vi "master_python_v1.0.vi"() -> ()   [LabVIEW 2026]
uses:
  Nanostage/Madlib.dll
  <vilib>/Utility/error.llb/DialogType.ctl
  <vilib>/DAQmx/read.llb/DAQmx Read (Analog 1D Wfm NChan NSamp).vi
  <vilib>/DAQmx/read.llb/DAQmx Read (Analog 1D Wfm NChan NSamp Duration).vi
  <vilib>/DAQmx/write.llb/DAQmx Write (Analog 2D DBL NChan NSamp).vi
  <vilib>/Utility/inputDevices.llb/keyboardAcquire.vi
panel:
  out "PID output":dbl format="%.2f"
  out "Setpoint":dbl
  in  "PID gains":T1={"proportional gain (Kc)"=0.5, "integral time (Ti, min)"=0.0, "derivative time (Td, min)"=0.0} {"derivative time (Td, min)" min=-1e-18 max=1000000000000000.0 step=1e-05 format="%.3f"; "integral time (Ti, min)" min=-1e-18 step=1e-05 format="%.6f"; "proportional gain (Kc)" min=-1e-18 step=1e-05 format="%.5f"}
  in  "output range":cluster{"output high":dbl, "output low":dbl}={"output high"=0.1, "output low"=-0.1} {"output low" format="%.2f"; "output high" format="%.2f"}
  in  "dt (s)":dbl=-1.0 format="%.3f"
  out "QPD":dbl
  out "Pos 0":dbl
  in  "Comment":string
  out "loop iteration":i32
  out "x start":dbl
  out "y start":dbl
  out "z start":dbl
  out "start iteration":dbl
  out "data":waveform(dbl)[](array[waveform])
  out "Numeric 2":i32
  out "Numeric":i32
  out "stop Ind":bool
  in  "Tab Control":enum32{"Main Control", "Calibration"}(tab)
  in  "Apply Force":bool
  out "Waveform Chart 6":waveform(dbl)(graph)
  out "Waveform Chart 5":waveform(dbl)(graph)
  in  "stop":bool
  in  "Record Data":bool
  in  "New File?":bool caption="new_file"
  out "QPD Position":cluster{"Array":dbl[], "Array":dbl[]}(graph)
  out "MT channels":waveform(dbl)[](graph)
  out "QPD Precise Position":cluster{"Array":dbl[], "Array":dbl[]}(graph)
  out "QPD Sum (Volt)":waveform(dbl)(graph)
  out "x":dbl
  out "y":dbl
  out "z":dbl
  in  "<":bool
  in  ">":bool
  in  "v":bool
  in  "^":bool
  in  "Down":bool
  in  "Up":bool
  in  "Fine":dbl=50.0
  in  "Step Size (nm)":bool
  in  "Course":dbl=500.0
  in  "Enable\ntapping":bool
  in  "DELAY (ms)":u32=10
  in  "x amplitude\n(um)":dbl
  in  "speed":i32=1
  in  "z amplitude (um)":dbl
  out "# oscillations":dbl
  in  "y amplitude\n(um)":dbl min=-25.0 max=25.0 step=0.05
  in  "Samples":u16=100 min=1 step=1
  in  "Centre":bool
  in  "Power Spectrum":bool
  in  "Duration (s)":dbl=2.0
  in  "Boolean":bool
  in  "Frequency":dbl=1.0 min=0.0 max=100.0 step=0.01
  in  "Amplitude":dbl=0.5 min=0.1 max=0.9 step=0.1
  in  "# Cycles":dbl=50.0 min=0.0 max=10000.0 step=0.001
  in  "Start Signal\nGen":bool
  in  "Desired Force (pN)":dbl step=0.01
  out "Measured Force (pN)":dbl(slide) scale=-2.0..2.0
  in  "Save Spectrum":bool
  in  "#":i32=1
  out "QPD nLR":waveform(dbl)(graph)
  out "QPD nBT":waveform(dbl)(graph)
  in  "Filename":path=path "C:/Users/localadmin/Desktop/220601 beadscan/7umscan2umbead.lvm"
  in  "Set 0 pN Position":bool
  out "QPD0":dbl
  in  "reinitialize?":bool
  in  "Conversion factor (pN/V)":dbl=1.0
  # "Left= anticlockwise"
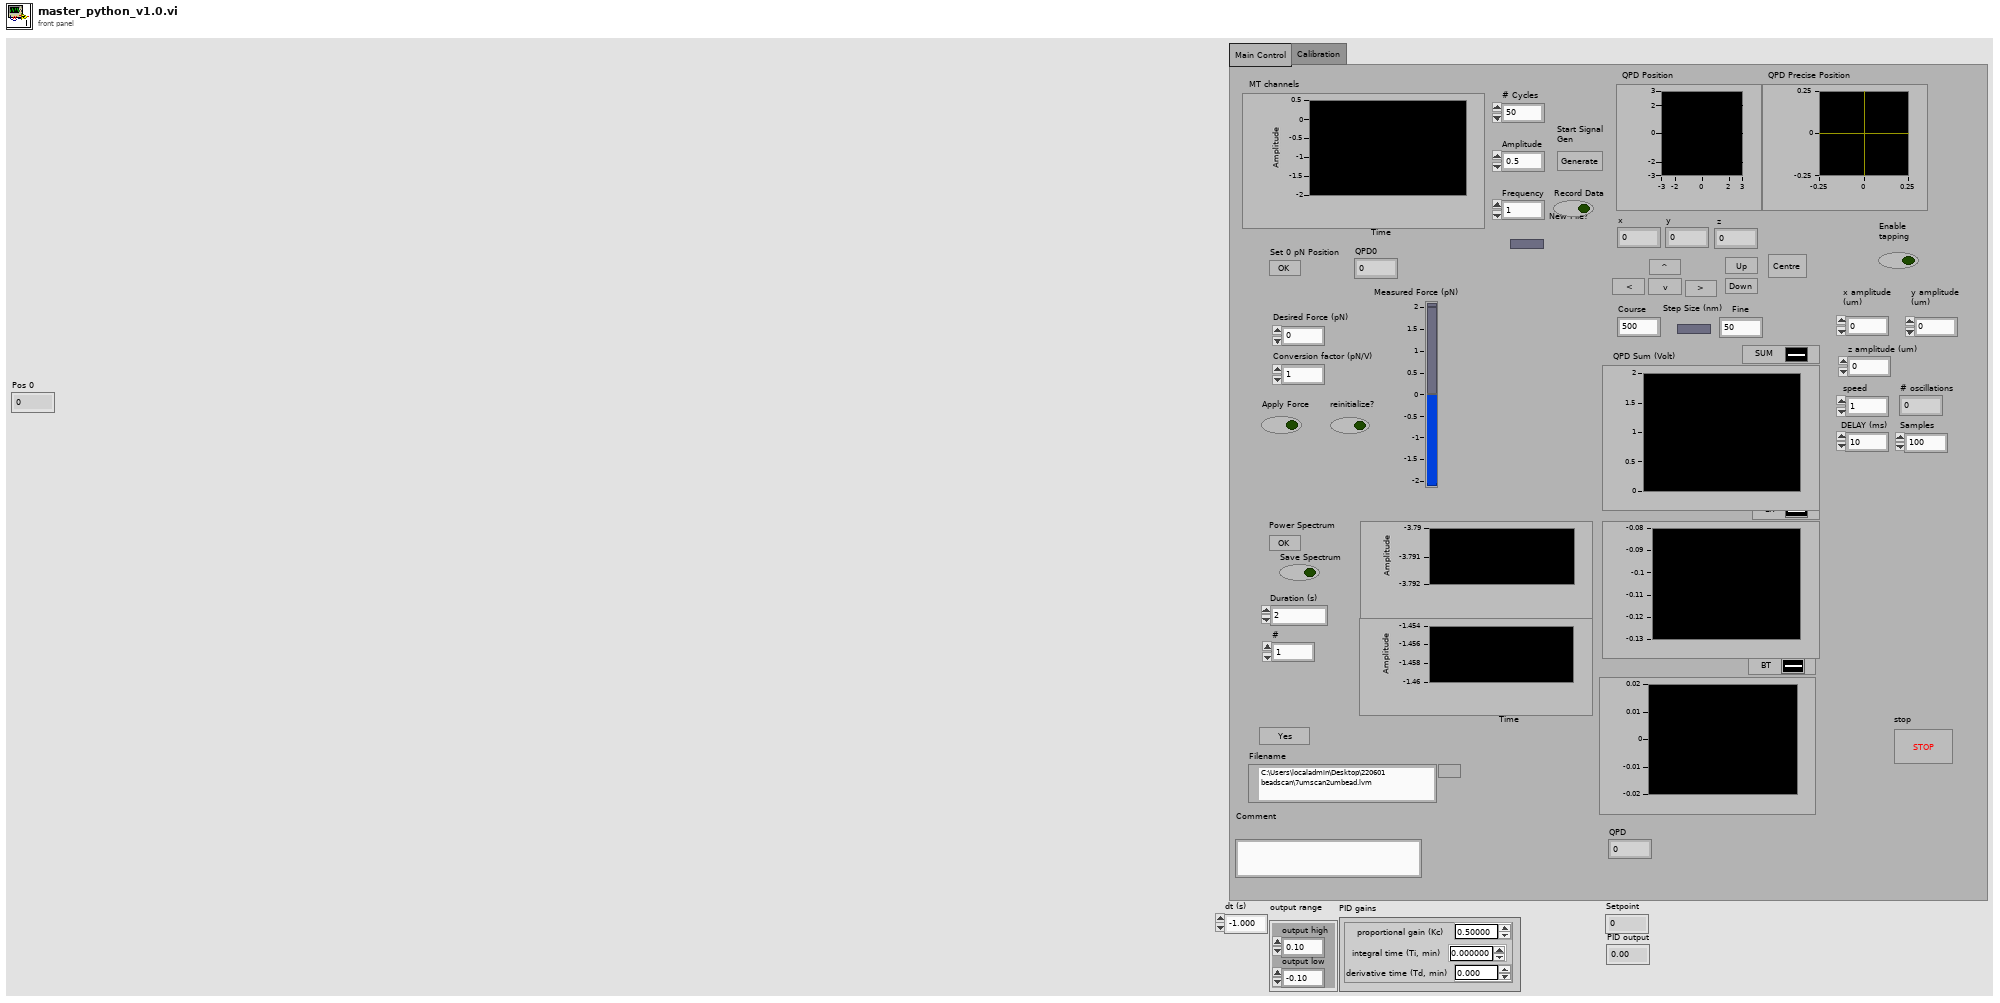
[diagram p1: front panel]
types:
  T1 = cluster{"proportional gain (Kc)":dbl, "integral time (Ti, min)":dbl, "derivative time (Td, min)":dbl}
  T2 = typedef "DialogType.ctl" = u16
  T3 = enum16{"Centre", "Move", "Tapping", "Calibration"}
  T4 = cluster{"kp":dbl, "ti":dbl, "td":dbl, "index":i32, "process_variable":dbl, "derivative_action":dbl, "integrated_error":dbl, "error":dbl, "output":dbl}
  T5 = enum16{"0", "1", "2", "3", "4", "5", "6", "7", "8", "9", "A", "B", "C", "D", "E", "F", "G", "H", "I", "J", "K", "L", "M", "N", "O", "P", "Q", "R", "S", "T", "U", "V", "W", "X", "Y", "Z", "F1", "F2", "F3", "F4", "F5", "F6", "F7", "F8", "F9", "F10", "F11", "F12", "F13", "F14", "F15", "ADD", "BACK", "BACKSLASH", "CAPITAL", "COMMA", "DECIMAL", "DELETE", "DIVIDE", "DOWN", "END", "EQUALS", "ESCAPE", "GRAVE (`)", "HOME", "INSERT", "LBRACKET", "LCONTROL", "LEFT", "L ALT", "LSHIFT", "LWIN", "MINUS", "MULTIPLY", "NEXT", "NUMLOCK", "NUMPAD_0", "NUMPAD_1", "NUMPAD_2", "NUMPAD_3", "NUMPAD_4", "NUMPAD_5", "NUMPAD_6", "NUMPAD_7", "NUMPAD_8", "NUMPAD_9", "PAUSE", "PERIOD", "PRIOR (PG UP)", "RBRACKET", "RCONTROL", "RETURN", "RIGHT", "R ALT", "RSHIFT", "RWIN", "SCROLL", "SEMICOLON", "SLASH", "SPACE", "SUBTRACT", "TAB", "UP", "ENTER (num pad)", "' (quote)"}[]
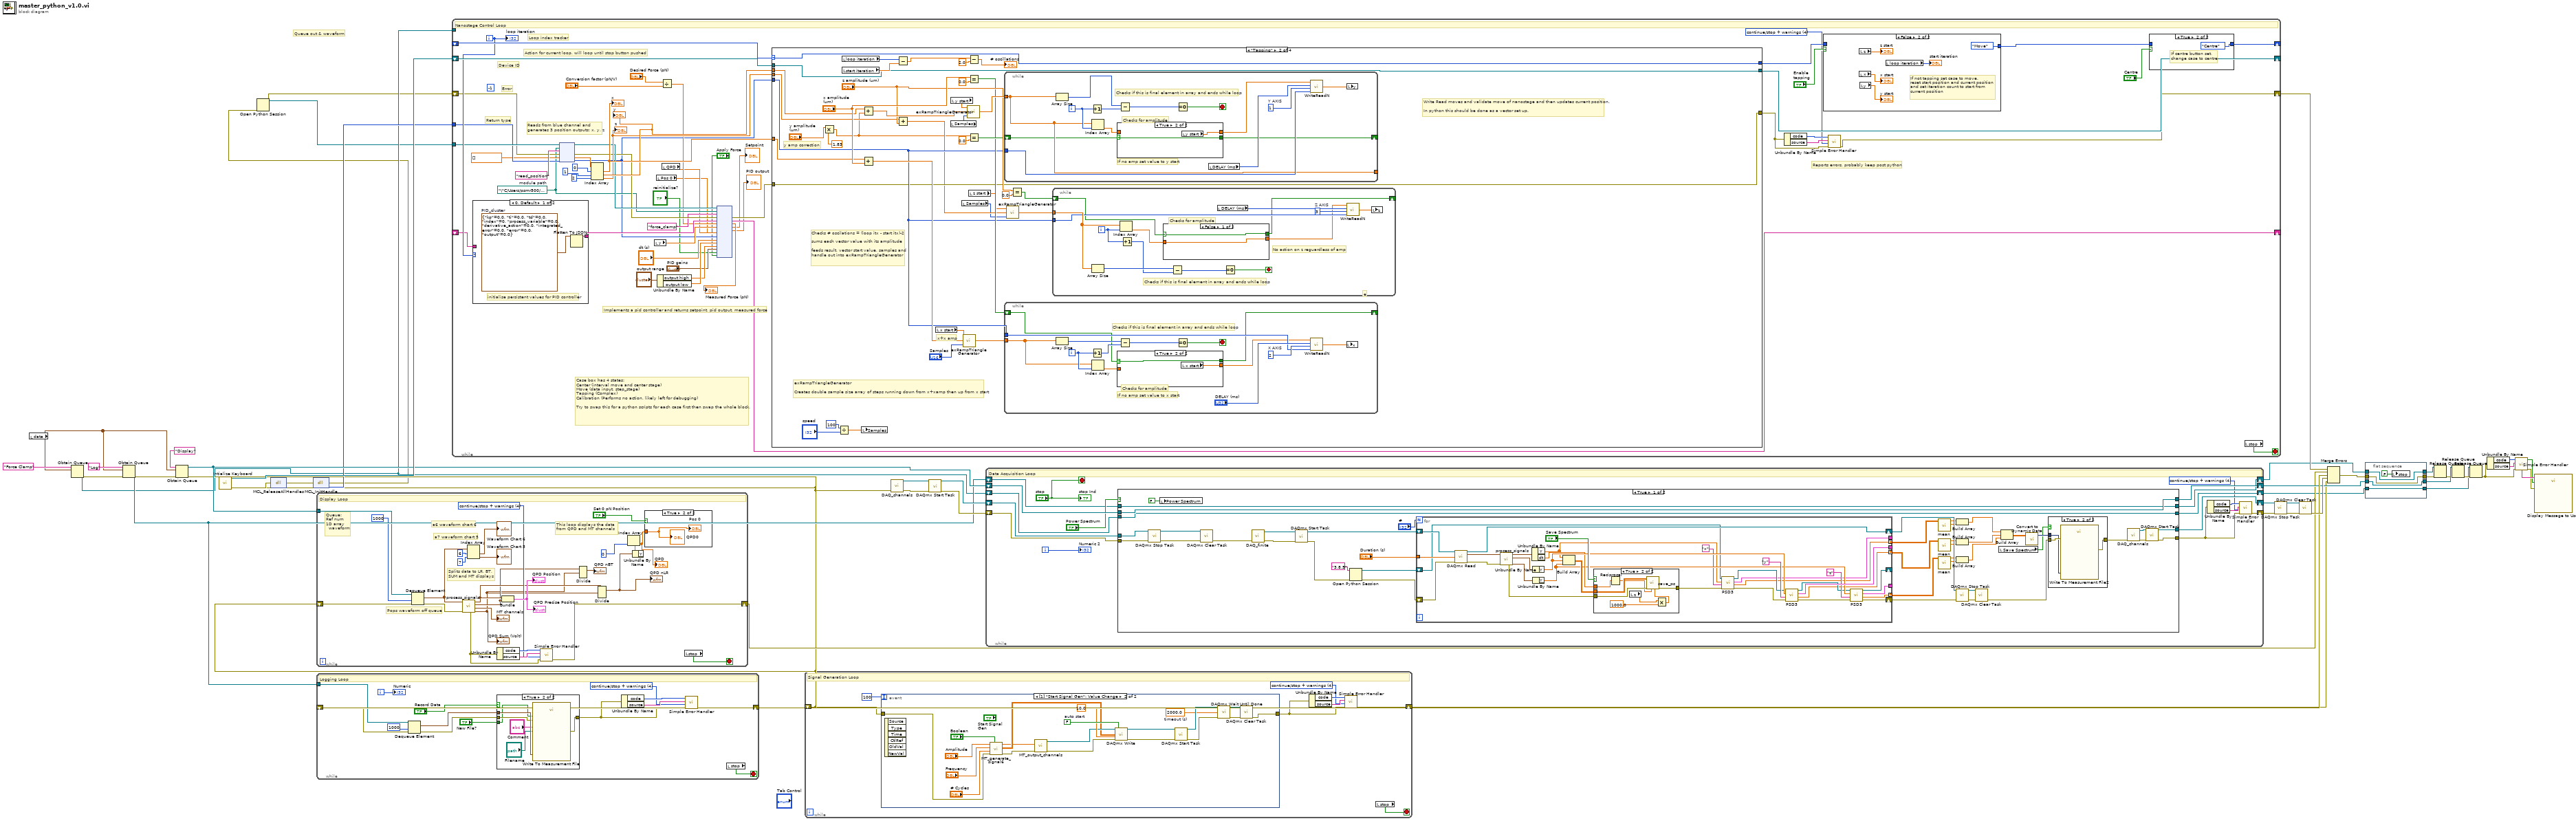
[diagram p0: block diagram]
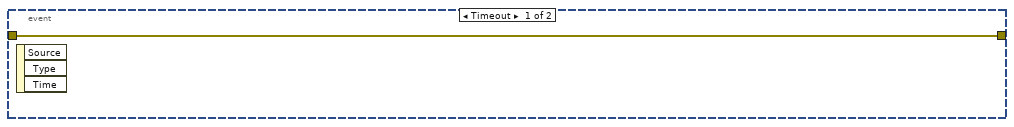
[diagram p2: hidden frame]
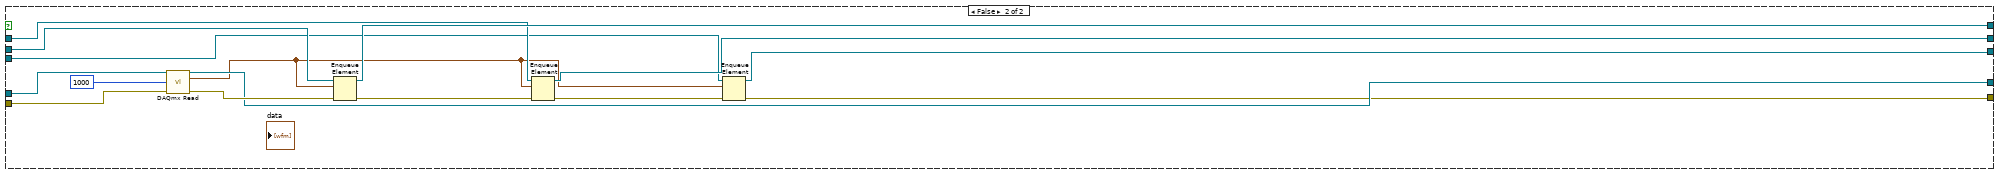
[diagram p5: hidden frame]
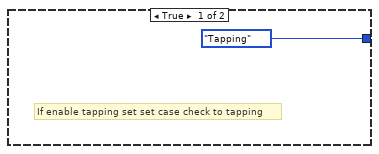
[diagram p9: hidden frame]
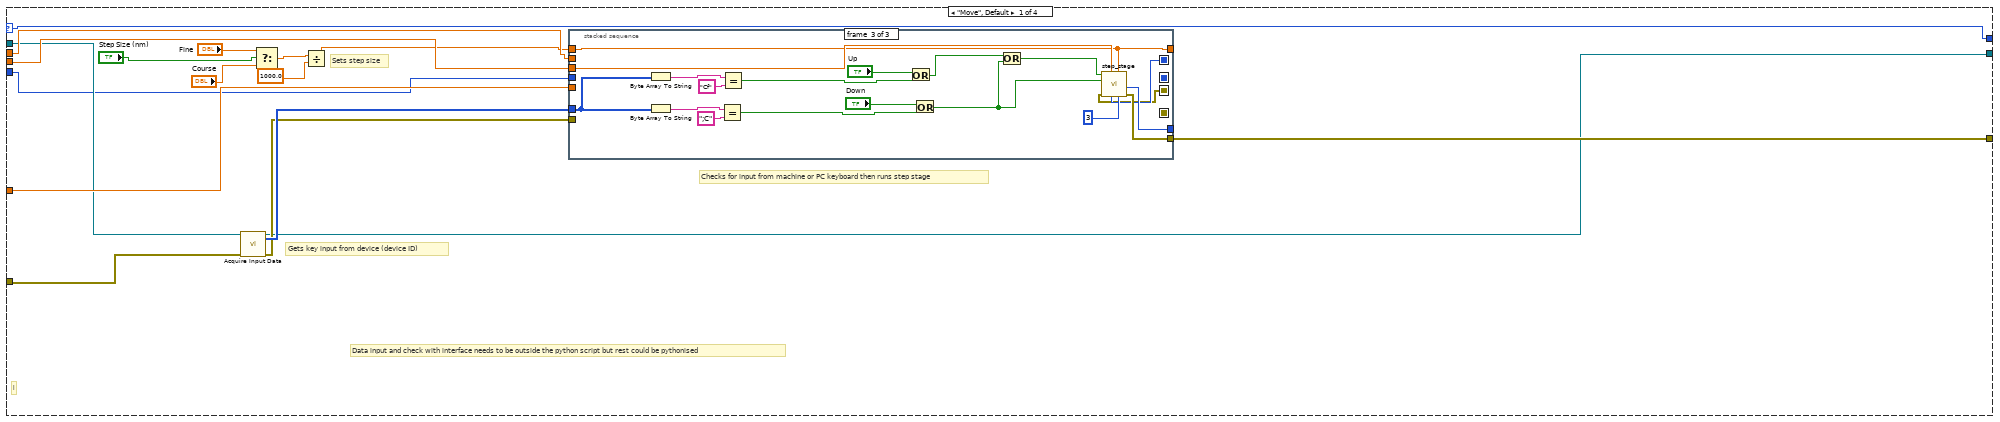
[diagram p10: hidden frame]
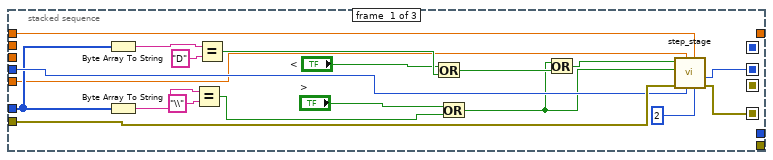
[diagram p11: hidden frame]
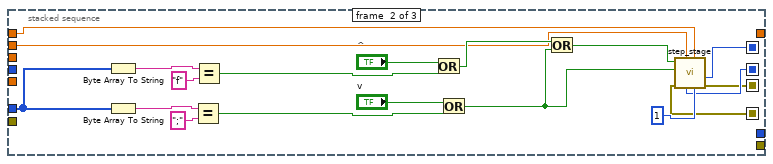
[diagram p12: hidden frame]
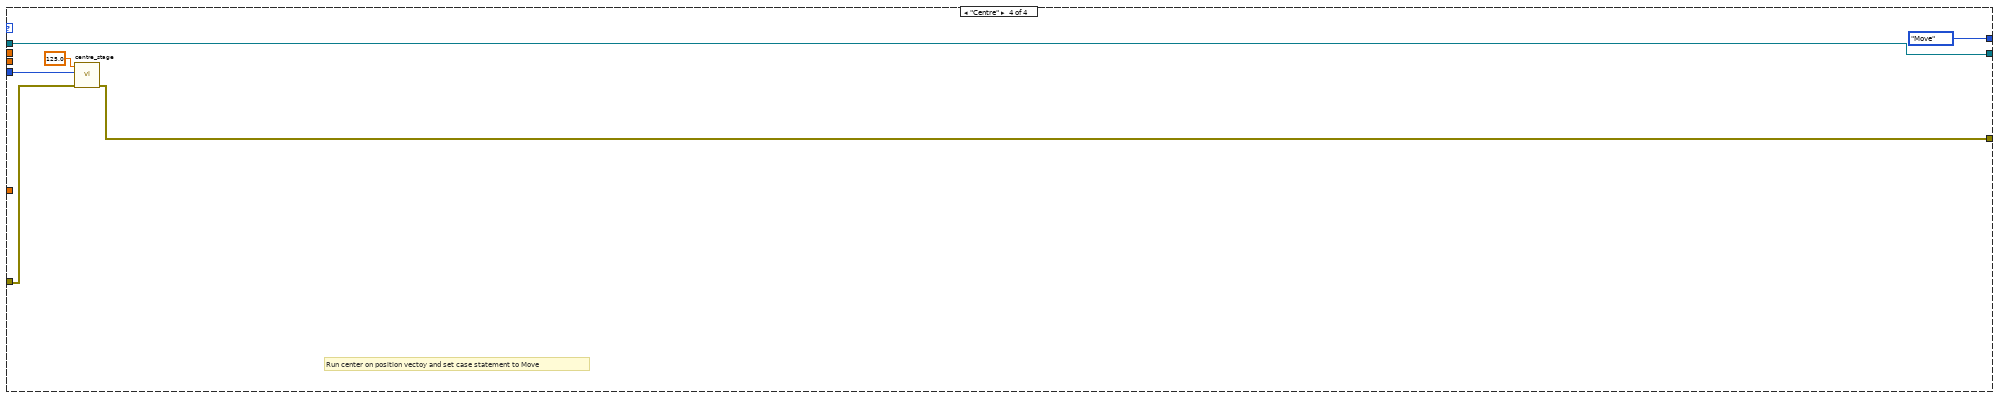
[diagram p17: hidden frame]
diagram:
  # "Queue out & waveform"
  n1 = local read "data"() -> (w9:waveform(dbl)[])
  n2 = Obtain Queue(name (unnamed)="Force Clamp", element data type=w9) -> (queue out=w4:refnum<queue>, error out=w11:errorcluster)  [unwired: 3 in, 1 out]
  n3 = Obtain Queue(name (unnamed)="Log", element data type=w9, error in (no error)=w11) -> (queue out=w15:refnum<queue>, error out=w20:errorcluster)  [unwired: 2 in, 1 out]
  n4 = Obtain Queue(name (unnamed)="Display", element data type=w9, error in (no error)=w20) -> (queue out=w22:refnum<queue>, error out=w13:errorcluster)  [unwired: 2 in, 1 out]
  n5 = call <vilib>:"Intialize Keyboard.vi"("error in (no error)"=w13) -> ("error out"=w25:errorcluster, "device ID"=w24:refnum<k1>)  [unwired: 9 out]
  n6 = dll-call lib="C:/Users/psmr500/PycharmProjects/COMBI-Tweez/LabVIEW Microscope Control/Nanostage/MADLib.dll" fn="MCL_ReleaseAllHandles"(error in=w25) -> (error out=w26:errorcluster)  [unwired: 3 in, 1 out]
  n7 = dll-call lib="C:/Users/psmr500/PycharmProjects/COMBI-Tweez/LabVIEW Microscope Control/Nanostage/MADLib.dll" fn="MCL_InitHandle"(error in=w26) -> (error out=w1:errorcluster, "return type"=w14:i32)  [unwired: 2 in, 1 out]
  n8 = Open Python Session(3:w1) -> (session out=w3:refnum<k35>, error out=w2:errorcluster)  [unwired: 2 in]
  n9 = while {
    tunnel: w22 -> [w72]
    shift-right: [w57] -> w28
    shift-left: w13 -> [w71]
    stop <- w70 stop-if-true
    w56 = T2 4 items=["no dialog", "OK message", "continue or stop message", "OK message + warnings", "continue/stop + warnings"] ("type of dialog (OK msg:1)")
    # "a7 waveform chart 5"
    # "a6 waveform chart 6"
    # "Splits data to LR, BT,\nSUM and MT displays"
    # "Pops waveform off queue"
    # "Queue:\nRef num\n1D array\n  waveform"
    # "This loop displays the data from QPD and MT channels"
    # "Display Loop"
    n10 = Dequeue Element(queue=w72, timeout in ms (-1)=1000, error in (no error)=w71) -> (element=w62:waveform(dbl)[], error out=w64:errorcluster)  [unwired: 2 out]
    n11 = call "process_signals.vi"("error in (no error)"=w64, "data"=w62) -> ("SUM"=w52:waveform(dbl), "MT"=→"MT channels":waveform(dbl)[], "BT"=w53:waveform(dbl), "LR"=w54:waveform(dbl), "error out"=w65:errorcluster)  [unwired: 5 in]
    "QPD Sum (Volt)" <- w52
    n12 = Index Array(array=w62, index #1=6 ("index"), index #2=7 ("index")) -> (element #1=→"Waveform Chart 6":waveform(dbl), element #2=→"Waveform Chart 5":waveform(dbl))
    n13 = Unbundle By Name(w65) -> ("code"=w67:i32, "source"=w66:string)
    n14 = Bundle("LR"=w54, "BT"=w53) -> (→"QPD Position" →"QPD Precise Position":cluster{"LR":waveform(dbl), "BT":waveform(dbl)})  [unwired: 1 in]
    n15 = call <vilib>:"Simple Error Handler.vi"("error code (no error:0)"=w67, "error source (\" \")"=w66, "type of dialog (OK msg:1)"=w56, "error in (no error)"=w65) -> ("error out"=w57:errorcluster)  [unwired: 1 in, 4 out]
    n16 = Divide(1:w52, 2:w53) -> (0:→"QPD nBT":waveform(dbl))  [unwired: 1 in, 1 out]
    n17 = Divide(1:w52, 2:w54) -> (0:w49:waveform(dbl))  [unwired: 1 in, 1 out]
    "QPD nLR" <- w49
    n18 = Unbundle By Name(w49) -> ("Y"=w50:dbl[])
    n19 = Index Array(array=w50, index=0) -> (element=w47:dbl)
    "QPD" <- w47
    n20 = case shown="True" "Set 0 pN Position" {
      tunnel: w47 -> [_ w73]
      frame False {
      }
      frame True {
        "Pos 0" <- w73
        "QPD0" <- w73
      }
    }
    n21 = local read "stop"() -> (w70:bool)
  }
  n22 = while {
    shift-right: [w75] -> w32
    shift-left: w13 -> [w87]
    tunnel: w15 -> [w86]
    i -> [w81]
    stop <- w76 stop-if-true
    w74 = T2 4 items=["no dialog", "OK message", "continue or stop message", "OK message + warnings", "continue/stop + warnings"] ("type of dialog (OK msg:1)")
    # "Logging Loop"
    n23 = Dequeue Element(queue=w86, timeout in ms (-1)=1000, error in (no error)=w87) -> (element=w83:waveform(dbl)[], error out=w84:errorcluster)  [unwired: 2 out]
    n24 = case shown="True" "Record Data" {
      tunnel: [w88 w94] -> w77
      tunnel: w83 -> [_ w93]
      tunnel: "New File?" -> [_ w90]
      tunnel: w84 -> [w88 w92]
      frame False {
      }
      frame True {
        n25 = call "Write To Measurement File"("Signals"=w93, "new_file"=w90, "error in (no error)"=w92, "Filename"="Filename", "Comment"="Comment") -> ("error out"=w94:errorcluster)  [unwired: 12 in, 2 out]
      }
    }
    n26 = Unbundle By Name(w77) -> ("code"=w79:i32, "source"=w78:string)
    n27 = call <vilib>:"Simple Error Handler.vi"("error code (no error:0)"=w79, "error source (\" \")"=w78, "type of dialog (OK msg:1)"=w74, "error in (no error)"=w77) -> ("error out"=w75:errorcluster)  [unwired: 1 in, 4 out]
    n28 = local read "stop"() -> (w76:bool)
    "Numeric" <- w81
  }
  n29 = while {
    shift-right: [w135] -> w23
    shift-left: w2 -> [w126]
    shift-right: [w140] -> _
    shift-left: w24 -> [w142]
    shift-right: [w136] -> _
    shift-left: _ -> [w141]
    tunnel: w14 -> [w125]
    tunnel: w4 -> [_]
    shift-right: [w110] -> _
    shift-left: _ -> [w129]
    tunnel: w3 -> [w127]
    i -> [w130]
    stop <- w146 stop-if-true
    w113 = path "/\"C/Users/psmr500/PycharmProjects/COMBI-Tweez/LabVIEW Microscope Control/Nanostage/nanostage.py\""  # module path
    (unwired) -1 ("timeout in ms (-1)")
    w134 = T2 4 items=["no dialog", "OK message", "continue or stop message", "OK message + warnings", "continue/stop + warnings"] ("type of dialog (OK msg:1)")
    # "Reports errors, probably keep post python"
    # "Case box has 4 states:\nCenter (interval move and center stage)\nMove (data input, step_stage)\nTapping (Complex)\nCalibration (Performs no action, likely left for debugging)\n\nTry to swap this for a python scripts for each case first then swap the whole block."
    # "Action for current loop, will loop until stop button pushed"
    # "Implements a pid controller and returns setpoint, pid output, measured force"
    # "Return type"
    # "Device ID"
    # "Error"
    # "Reads from blue channel and \ngenerates 3 position outputs: x, y, z"
    # "Loop index tracker"
    # "Nanostage Control Loop"
    n30 = case shown="0, Default" w130 {
      tunnel: [w147 w149] -> w111
      tunnel: w129 -> [_ w149]
      frame 0, Default {
        w148 = T4 {"kp"=0.0, "ti"=0.0, "td"=0.0, "index"=0, "process_variable"=0.0, "derivative_action"=0.0, "integrated_error"=0.0, "error"=0.0, "output"=0.0}  # PID_cluster
        # "initialise persistent values for PID controller"
        n31 = Flatten To JSON(anything=w148) -> (JSON string=w147:string)  [unwired: 2 in, 1 out]
      }
      frame 1 {
      }
    }
    n32 = node(w127, w113, "read_position" ("function name"), w126, dbl[] [], w125) -> (w116:refnum<k35>, w115:errorcluster, w123:dbl[], w105:i32)  [unwired: 2 out]
    n33 = Index Array(array=w123, index #1=0 ("index"), index #2=1 ("index"), index #3=2 ("index")) -> (element #1=w119:dbl, element #2=w118:dbl, element #3=w117:dbl)
    "x" <- w119
    "y" <- w118
    "z" <- w117
    n34 = local read "y"() -> (w108:dbl)
    n35 = local read "Pos 0"() -> (w106:dbl)
    n36 = Unbundle By Name("output range") -> ("output high"=w101:dbl, "output low"=w102:dbl)
    n37 = Divide(x="Desired Force (pN)", y="Conversion factor (pN/V)") -> (x/y=w109:dbl)
    n38 = local read "QPD"() -> (w107:dbl)
    n39 = node(w116, w113, "force_clamp" ("function name"), w115, w111, w109, w108, w107, w106, w105, "dt (s)", w102, w101, "PID gains", "reinitialize?", "Apply Force") -> (w114:errorcluster, w110:string, →"Measured Force (pN)":dbl, →"Setpoint":dbl, →"PID output":dbl)  [unwired: 8 in, 3 out]
    n40 = case shown="\"Tapping\"" w141 {
      selector: w141 -> [w158 w242 w333 _]
      tunnel: w114 -> [w164 w244 w331 w348]
      tunnel: w105 -> [w162 w245 w332 w347]
      tunnel: [w160 w244 w325 w346] -> w143
      tunnel: w119 -> [w174 w247 w335 _]
      tunnel: w118 -> [w173 w246 w334 _]
      tunnel: w117 -> [w172 w241 _ _]
      tunnel: w142 -> [w165 w243 w324 w343]
      tunnel: [w158 w242 w333 T3."Move"] -> w139
      tunnel: [w159 w243 w324 w343] -> w140
      frame "Move", Default {
        # "Data input and check with interface needs to be outside the python script but rest could be pythonised"
        # "Checks for input from machine or PC keyboard then runs step stage"
        # "Sets step size"
        # "Gets key input from device (device ID)"
        # "l"
        n41 = call-poly <vilib>:"Acquire Input Data.vi"("device ID"=w165, "error in (no error)"=w164) -> ("device ID"=w159:refnum<k1>, "keys pressed"=w163:T5, "error out"=w161:errorcluster)  [unwired: 15 out]
        n42 = Select(t="Fine", s="Step Size (nm)", f="Course") -> (s? t:f=w168:dbl)
        n43 = Divide(x=w168, y=1000.0) -> (x/y=w166:dbl)
        n44 = stacked-sequence {
          seq-local: [w190 _ _] -> [_ w211 _]
          seq-local: [w189 _ _] -> [_ w210 _]
          seq-local: [_ w208 _] -> [_ _ w227]
          seq-local: [_ w209 _] -> [_ _ w226]
          tunnel: w161 -> [w193 _ _]
          tunnel: w162 -> [w192 _ _]
          tunnel: w174 -> [w176 _ _]
          tunnel: w173 -> [_ w195 _]
          tunnel: w172 -> [_ _ w230]
          tunnel: [_ _ w228] -> w160
          tunnel: [_ _ w229] -> _
          tunnel: w163 -> [w178 w197 w214]
          tunnel: [_ _ w213] -> _
          tunnel: w166 -> [w177 w196 w213]
          frame #0 {
            n45 = Byte Array To String(unsigned byte array=w178) -> (string=w186:string)
            n46 = Byte Array To String(unsigned byte array=w178) -> (string=w188:string)
            n47 = Equal?(x=w188, y="\\") -> (x = y?=w184:bool)
            n48 = Equal?(x=w186, y="D") -> (x = y?=w183:bool)
            n49 = Or(x="<", y=w183) -> (x .or. y?=w180:bool)
            n50 = Or(x=">", y=w184) -> (x .or. y?=w175:bool)
            n51 = Or(x=w175, y=w180) -> (x .or. y?=w179:bool)
            n52 = call "step_stage.vi"("axis"=u32 2, "step"=w177, "handle"=w192, "position"=w176, "error in"=w193, "+/-"=w175, "move"=w179) -> ("error out"=w189:errorcluster, "handle out"=w190:i32)  [unwired: 3 in]
          }
          frame #1 {
            n53 = Byte Array To String(unsigned byte array=w197) -> (string=w207:string)
            n54 = Byte Array To String(unsigned byte array=w197) -> (string=w205:string)
            n55 = Equal?(x=w205, y=";") -> (x = y?=w200:bool)
            n56 = Equal?(x=w207, y="f") -> (x = y?=w203:bool)
            n57 = Or(x="^", y=w203) -> (x .or. y?=w199:bool)
            n58 = Or(x="v", y=w200) -> (x .or. y?=w198:bool)
            n59 = Or(x=w199, y=w198) -> (x .or. y?=w194:bool)
            n60 = call "step_stage.vi"("axis"=u32 1, "step"=w196, "handle"=w211, "position"=w195, "error in"=w210, "+/-"=w198, "move"=w194) -> ("error out"=w209:errorcluster, "handle out"=w208:i32)  [unwired: 3 in]
          }
          frame #2 {
            n61 = Byte Array To String(unsigned byte array=w214) -> (string=w225:string)
            n62 = Byte Array To String(unsigned byte array=w214) -> (string=w223:string)
            n63 = Equal?(x=w223, y=";C") -> (x = y?=w220:bool)
            n64 = Equal?(x=w225, y="Cf") -> (x = y?=w221:bool)
            n65 = Or(x="Up", y=w221) -> (x .or. y?=w219:bool)
            n66 = Or(x="Down", y=w220) -> (x .or. y?=w217:bool)
            n67 = Or(x=w219, y=w217) -> (x .or. y?=w218:bool)
            n68 = call "step_stage.vi"("axis"=u32 3, "step"=w213, "handle"=w227, "position"=w230, "error in"=w226, "+/-"=w217, "move"=w218) -> ("error out"=w228:errorcluster, "handle out"=w229:i32)  [unwired: 3 in]
          }
        }
      }
      frame "Tapping" {
        # "Write Read moves and validate move of nanostage and then updates current position.\n\nIn python this should be done as a vector set up."
        # "exRampTriangleGenerator\n\nCreates double sample size array of steps running down from x+xamp then up from x start"
        # "Checks # oscilations = (loop itx - start itx)-2\n\nsums each vector value with its amplitude\n\nfeeds result, vector start value, samples and \nhandle out into exRampTriangleGenerator"
        # "x+x amp"
        # "y amp correction"
        n69 = Multiply(x="y amplitude\n(um)", y=1.83) -> (x*y=w233:dbl)
        n70 = Divide(x=100, y="speed") -> (x/y=w264:dbl)
        n71 = local read "loop iteration"() -> (w259:i32)
        n72 = local read "start iteration"() -> (w260:dbl)
        n73 = local write "Samples"(w264) -> ()
        n74 = Add(x=w246, y=w233) -> (x+y=w263:dbl)
        n75 = Add(x=w247, y="x amplitude\n(um)") -> (x+y=w268:dbl)
        n76 = Subtract(x=w259, y=w260) -> (x-y=w258:dbl)
        n77 = Add(x=w241, y="z amplitude (um)") -> (x+y=w240:dbl)
        n78 = local read "x start"() -> (w237:dbl)
        n79 = local read "Samples"() -> (w261:u16)
        n80 = local read "y start"() -> (w235:dbl)
        n81 = local read "Samples"() -> (w239:u16)
        n82 = call "exRampTriangleGenerator.vi"("Number of positions"="Samples", "End(um)"=w268, "Start(um)"=w237) -> ("Array"=w269:dbl[])
        n83 = call "exRampTriangleGenerator.vi"("Number of positions"=w261, "End(um)"=w263, "Start(um)"=w235) -> ("Array"=w262:dbl[])
        n84 = Subtract(x=w258, y=2.0) -> (x-y=→"# oscillations":dbl)
        n85 = Equal?(x="x amplitude\n(um)", y=0.0) -> (x = y?=w249:bool)
        n86 = Equal?(x=w233, y=0.0) -> (x = y?=w250:bool)
        n87 = local read "z start"() -> (w236:dbl)
        n88 = while {
          tunnel: [w293] -> _
          tunnel: w245 -> [w300]
          tunnel: w262 -> [w293]
          shift-right: [w289] -> _
          shift-left: w250 -> [w290]
          i -> [w301]
          stop <- w295 stop-if-true
          w296 = 1  # Y AXIS
          # "If no amp set value to y start"
          # "Checks if this is final element in array and ends while loop"
          # "Checks for amplitude"
          n89 = Array Size(array=w293) -> (size(s)=w298:i32)
          n90 = Increment(x=w301) -> (x+1=w297:i32)
          n91 = Index Array(array=w293, index=w301) -> (element=w292:dbl)
          n92 = case shown="True" w290 {
            selector: w290 -> [w302 w305]
            tunnel: w292 -> [w303 _]
            tunnel: [w303 w304] -> w291
            tunnel: [w302 w305] -> w289
            frame False {
            }
            frame True {
              n93 = local read "y start"() -> (w304:dbl)
            }
          }
          n94 = Subtract(x=w298, y=w297) -> (x-y=w299:i32)
          n95 = Equal To 0?(x=w299) -> (x = 0?=w295:bool)
          n96 = local read "DELAY (ms)"() -> (w294:u32)
          n97 = call "WriteReadN.vi"("Handle"=w300, "Axis"=w296, "Delay (ms)"=w294, "Move to (um)"=w291) -> ("Current Position (um)"=w288:dbl)
          n98 = local write "y"(w288) -> ()
        }
        n99 = while {
          tunnel: w269 -> [w311]
          tunnel: w245 -> [w312]
          shift-right: [w307] -> _
          shift-left: w249 -> [w308]
          i -> [w315]
          stop <- w317 stop-if-true
          w313 = 2  # X AXIS
          # "If no amp set value to x start"
          # "Checks if this is final element in array and ends while loop"
          # "Checks for amplitude"
          n100 = Array Size(array=w311) -> (size(s)=w318:i32)
          n101 = Increment(x=w315) -> (x+1=w316:i32)
          n102 = Index Array(array=w311, index=w315) -> (element=w310:dbl)
          n103 = case shown="True" w308 {
            selector: w308 -> [w320 w323]
            tunnel: w310 -> [w321 _]
            tunnel: [w321 w322] -> w309
            tunnel: [w320 w323] -> w307
            frame False {
            }
            frame True {
              n104 = local read "x start"() -> (w322:dbl)
            }
          }
          n105 = Subtract(x=w318, y=w316) -> (x-y=w319:i32)
          n106 = Equal To 0?(x=w319) -> (x = 0?=w317:bool)
          n107 = call "WriteReadN.vi"("Handle"=w312, "Axis"=w313, "Delay (ms)"="DELAY (ms)", "Move to (um)"=w309) -> ("Current Position (um)"=w306:dbl)
          n108 = local write "x"(w306) -> ()
        }
        n109 = call "exRampTriangleGenerator.vi"("Number of positions"=w239, "End(um)"=w240, "Start(um)"=w236) -> ("Array"=w238:dbl[])
        n110 = Equal?(x="z amplitude (um)", y=0.0) -> (x = y?=w248:bool)
        n111 = while {
          tunnel: w238 -> [w276]
          tunnel: w245 -> [w275]
          shift-right: [w271] -> _
          shift-left: w248 -> [w272]
          i -> [w279]
          stop <- w281 stop-if-true
          w278 = 3  # Z AXIS
          # "No action on z reguardless of amp"
          # "Checks if this is final element in array and ends while loop"
          # "Checks for amplitude"
          # "e"
          n112 = Array Size(array=w276) -> (size(s)=w282:i32)
          n113 = Index Array(array=w276, index=w279) -> (element=w274:dbl)
          n114 = Increment(x=w279) -> (x+1=w280:i32)
          n115 = case shown="False" w272 {
            selector: w272 -> [w284 w287]
            tunnel: w274 -> [w285 w286]
            tunnel: [w285 w286] -> w273
            tunnel: [w284 w287] -> w271
            frame False {
            }
            frame True {
            }
          }
          n116 = Subtract(x=w282, y=w280) -> (x-y=w283:i32)
          n117 = local read "DELAY (ms)"() -> (w277:u32)
          n118 = Equal To 0?(x=w283) -> (x = 0?=w281:bool)
          n119 = call "WriteReadN.vi"("Handle"=w275, "Axis"=w278, "Delay (ms)"=w277, "Move to (um)"=w273) -> ("Current Position (um)"=w270:dbl)
          n120 = local write "z"(w270) -> ()
        }
      }
      frame "Calibration" {
        n121 = flat-sequence {
          tunnel: w331 -> [w336]
          tunnel: [w336] -> w326
          tunnel: [w337] -> w327
          tunnel: w326 -> [w337]
          tunnel: w332 -> [_]
          tunnel: w335 -> [_]
          tunnel: w334 -> [_]
          tunnel: [w338] -> w328
          tunnel: w327 -> [w338]
          tunnel: [w339] -> w329
          tunnel: w328 -> [w339]
          tunnel: [w341] -> _
          tunnel: w332 -> [w341]
          tunnel: [w340] -> w330
          tunnel: w329 -> [w340]
          tunnel: w330 -> [w342]
          tunnel: [w342] -> w325
          frame #0 {
          }
          frame #1 {
          }
          frame #2 {
          }
          frame #3 {
          }
          frame #4 {
          }
          frame #5 {
          }
        }
      }
      frame "Centre" {
        # "Run center on position vectoy and set case statement to Move"
        n122 = call "centre_stage.vi"("error in"=w348, "handle in"=w347, "Destination"=125.0) -> ("error out"=w346:errorcluster)  [unwired: 7 in, 1 out]
      }
    }
    n123 = Unbundle By Name(w143) -> ("code"=w145:i32, "source"=w144:string)
    n124 = case shown="False" "Enable\ntapping" {
      tunnel: w139 -> [_ _]
      tunnel: [T3."Tapping" T3."Move"] -> w133
      frame True {
        # "If enable tapping set set case check to tapping"
      }
      frame False {
        # "If not tapping set case to move.\nreset start position and current position \nand set iteration count to start from \ncurrent position"
        n125 = local read "z"() -> (→"z start":dbl)
        n126 = local read "x"() -> (→"x start":dbl)
        n127 = local read "y"() -> (→"y start":dbl)
        n128 = local read "loop iteration"() -> (→"start iteration":i32)
      }
    }
    n129 = call <vilib>:"Simple Error Handler.vi"("error code (no error:0)"=w145, "error source (\" \")"=w144, "type of dialog (OK msg:1)"=w134, "error in (no error)"=w143) -> ("error out"=w135:errorcluster)  [unwired: 1 in, 4 out]
    n130 = case shown="True" "Centre" {
      tunnel: [w150 T3."Centre"] -> w136
      tunnel: w133 -> [w150 _]
      frame False {
        # "If not centre no effect"
      }
      frame True {
        # "If centre button set, \nchange case to centre"
      }
    }
    n131 = local read "stop"() -> (w146:bool)
    "loop iteration" <- w130
  }
  n132 = while {
    shift-right: [w350] -> w12
    shift-left: w13 -> [w355]
    stop <- w356 stop-if-true
    w351 = T2 4 items=["no dialog", "OK message", "continue or stop message", "OK message + warnings", "continue/stop + warnings"] ("type of dialog (OK msg:1)")
    # "Signal Generation Loop"
    n133 = event shown="[1] \"Start Signal Gen\": Value Change" {
      selector: _ -> [_ _]
      dyn-events: _ -> [_ _]
      timeout: 100 -> [_ _]
      tunnel: [w357 w360] -> w349
      tunnel: w355 -> [w357 w359]
      event Timeout {
        n134 = event-data() -> ()  [unwired: 1 in, 3 out]
      }
      event "Start Signal\nGen": Value Change {
        w369 = 2000.0  # timeout (s)
        w368 = FALSE  # auto start
        n135 = event-data() -> ()  [unwired: 1 in, 6 out]
        n136 = call "MT_generate_signal6.vi"("Direction"="Boolean", "error in (no error)"=w359, "# cycles"="# Cycles", "frequency"="Frequency", "amplitude"="Amplitude") -> ("error out"=w365:errorcluster, "signals out"=w363:dbl[][], "# samples"=w362:dbl)  [unwired: 4 in]
        n137 = call "MT_output_channels.vi"("error in"=w365, "number of samples"=w362) -> ("error out"=w364:errorcluster, "task out"=w366:refnum<k21>)  [unwired: 8 in]
        n138 = call-poly <vilib>:"DAQmx Write.vi"("task/channels in"=w366, "auto start"=w368, "data"=w363, "timeout"=10.0, "error in"=w364) -> ("task out"=w373:refnum<k21>, "error out"=w374:errorcluster)  [unwired: 8 in, 1 out]
        n139 = call <vilib>:"DAQmx Start Task.vi"("task/channels in"=w373, "error in"=w374) -> ("task out"=w370:refnum<k21>, "error out"=w371:errorcluster)  [unwired: 12 in]
        n140 = call <vilib>:"DAQmx Wait Until Done.vi"("task/channels in"=w370, "timeout (sec)"=w369, "error in"=w371) -> ("task out"=w375:refnum<k21>, "error out"=w372:errorcluster)  [unwired: 11 in]
        n141 = call <vilib>:"DAQmx Clear Task.vi"("task in"=w375, "error in"=w372) -> ("error out"=w360:errorcluster)  [unwired: 13 in]
      }
    }
    n142 = Unbundle By Name(w349) -> ("code"=w353:i32, "source"=w352:string)
    n143 = call <vilib>:"Simple Error Handler.vi"("error code (no error:0)"=w353, "error source (\" \")"=w352, "type of dialog (OK msg:1)"=w351, "error in (no error)"=w349) -> ("error out"=w350:errorcluster)  [unwired: 1 in, 4 out]
    n144 = local read "stop"() -> (w356:bool)
  }
  n145 = call "DAQ_channels.vi"("error in"=w13) -> ("error out"=w40:errorcluster, "task out"=w41:refnum<k21>)  [unwired: 9 in]
  n146 = call <vilib>:"DAQmx Start Task.vi"("task/channels in"=w41, "error in"=w40) -> ("task out"=w44:refnum<k21>, "error out"=w45:errorcluster)  [unwired: 12 in]
  n147 = while {
    shift-right: [w379] -> w39
    shift-left: w45 -> [w394]
    shift-right: [w391] -> w31
    shift-left: w22 -> [w392]
    shift-right: [w388] -> w27
    shift-left: w44 -> [w393]
    shift-right: [w383] -> w19
    shift-left: w15 -> [w382]
    shift-right: [w380] -> w5
    shift-left: w4 -> [w381]
    i -> [w389]
    stop <- "stop" stop-if-true
    w378 = T2 4 items=["no dialog", "OK message", "continue or stop message", "OK message + warnings", "continue/stop + warnings"] ("type of dialog (OK msg:1)")
    # "Data Acquisition Loop"
    n148 = case shown="True" "Power Spectrum" {
      tunnel: w394 -> [w436 w498]
      tunnel: w393 -> [w437 w496]
      tunnel: w392 -> [w435 w495]
      tunnel: [w435 w494] -> w391
      tunnel: [w422 w493] -> w388
      tunnel: [w421 w487] -> w384
      tunnel: w382 -> [w434 w491]
      tunnel: [w434 w489] -> w383
      tunnel: w381 -> [w419 w486]
      tunnel: [w419 w485] -> w380
      frame True {
        n149 = call <vilib>:"DAQmx Stop Task.vi"("task/channels in"=w437, "error in"=w436) -> ("task out"=w433:refnum<k21>, "error out"=w432:errorcluster)  [unwired: 12 in]
        n150 = local write "Power Spectrum"(FALSE ("Power Spectrum")) -> ()
        n151 = call <vilib>:"DAQmx Clear Task.vi"("task in"=w433, "error in"=w432) -> ("error out"=w418:errorcluster)  [unwired: 13 in]
        n152 = call "DAQ_finite.vi"("error in"=w418) -> ("error out"=w430:errorcluster, "task out"=w431:refnum<k21>)  [unwired: 9 in]
        n153 = call <vilib>:"DAQmx Start Task.vi"("task/channels in"=w431, "error in"=w430) -> ("task out"=w429:refnum<k21>, "error out"=w417:errorcluster)  [unwired: 12 in]
        n154 = Open Python Session(python version="3.8.5" ("Python version"), 3:w417) -> (session out=w414:refnum<k35>, error out=w416:errorcluster)  [unwired: 1 in]
        n155 = for {
          N: "#" -> [_]
          tunnel: "Duration (s)" -> [w472]
          tunnel: [w470] -> _
          tunnel: [w456] -> _
          tunnel: [w447] -> _
          shift-right: [w473] -> w425
          shift-left: w429 -> [w474]
          shift-right: [w454] -> _
          shift-left: w414 -> [w452]
          shift-right: [w458] -> w395
          shift-left: w416 -> [w446]
          tunnel: [w444] -> w413 mode=indexing
          tunnel: [w443] -> w412 mode=indexing
          tunnel: [w442] -> w411 mode=indexing
          n156 = call-poly <vilib>:"DAQmx Read.vi"("task/channels in"=w474, "duration"=w472, "error in"=w446) -> ("task out"=w473:refnum<k21>, "data"=w471:waveform(dbl)[], "error out"=w445:errorcluster)  [unwired: 10 in]
          n157 = call "process_signals.vi"("error in (no error)"=w445, "data"=w471) -> ("SUM"=w466:waveform(dbl), "BT"=w468:waveform(dbl), "LR"=w467:waveform(dbl), "error out"=w462:errorcluster)  [unwired: 5 in, 1 out]
          n158 = Unbundle By Name(w467) -> ("Y"=w448:dbl[], "dt"=w463:dbl)
          n159 = Unbundle By Name(w468) -> ("Y"=w465:dbl[])
          n160 = Unbundle By Name(w466) -> ("Y"=w457:dbl[])
          n161 = Build Array(w448, w465, w457) -> (w464:dbl[][])
          n162 = case shown="True" "Save Spectrum" {
            tunnel: w464 -> [_ w483]
            tunnel: w463 -> [_ w480]
            tunnel: w462 -> [w475 w482]
            tunnel: [w475 w481] -> w450
            frame False {
            }
            frame True {
              n163 = Reciprocal(x=w480) -> (1/x=w479:dbl)
              n164 = local read "z"() -> (w478:dbl)
              n165 = Multiply(x=w478, y=1000.0) -> (x*y=w477:dbl)
              n166 = call "save_ps.vi"("Height"=w477, "Rate"=w479, "error in"=w482, "QPD Data"=w483) -> ("error out"=w481:errorcluster)  [unwired: 7 in]
            }
          }
          n167 = call "PSD3.vi"("error in (no error)"=w450, "axis"="x", "data"=w448, "Refnum in"=w452) -> ("error out"=w449:errorcluster, "parameters"=w444:dbl[], "Array"=w447:cluster{dbl, dbl, dbl[]}[], "Refnum out"=w451:refnum<k35>)  [unwired: 4 in]
          n168 = call "PSD3.vi"("error in (no error)"=w449, "axis"="y", "data"=w465, "Refnum in"=w451) -> ("error out"=w459:errorcluster, "parameters"=w443:dbl[], "Array"=w470:cluster{dbl, dbl, dbl[]}[], "Refnum out"=w455:refnum<k35>)  [unwired: 4 in]
          n169 = call "PSD3.vi"("error in (no error)"=w459, "axis"="z", "data"=w457, "Refnum in"=w455) -> ("error out"=w458:errorcluster, "parameters"=w442:dbl[], "Array"=w456:cluster{dbl, dbl, dbl[]}[], "Refnum out"=w454:refnum<k35>)  [unwired: 4 in]
        }
        n170 = call "mean.vi"("parameters"=w413) -> ("k"=w406:dbl, "b"=w407:dbl)  [unwired: 9 in]
        n171 = call "mean.vi"("parameters"=w412) -> ("k"=w404:dbl, "b"=w405:dbl)  [unwired: 9 in]
        n172 = call "mean.vi"("parameters"=w411) -> ("k"=w402:dbl, "b"=w403:dbl)  [unwired: 9 in]
        n173 = Build Array(w407, w406) -> (w409:dbl[])
        n174 = Build Array(w405, w404) -> (w396:dbl[])
        n175 = Build Array(w403, w402) -> (w408:dbl[])
        n176 = call <vilib>:"DAQmx Stop Task.vi"("task/channels in"=w425, "error in"=w395) -> ("task out"=w427:refnum<k21>, "error out"=w426:errorcluster)  [unwired: 12 in]
        n177 = call <vilib>:"DAQmx Clear Task.vi"("task in"=w427, "error in"=w426) -> ("error out"=w401:errorcluster)  [unwired: 13 in]
        n178 = local read "Save Spectrum"() -> (w397:bool)
        n179 = Build Array(w409, w396, w408) -> (w399:dbl[][])
        n180 = call "Convert to Dynamic Data"("2D Array"=w399) -> ("Dynamic Data Type"=w398:dynamicdata)  [unwired: 3 in]
        n181 = case shown="True" w397 {
          tunnel: w401 -> [w438 w441]
          tunnel: [w438 w440] -> w400
          tunnel: w398 -> [_ w439]
          frame False {
          }
          frame True {
            n182 = call "Write To Measurement File2"("Signals"=w439, "error in (no error)"=w441) -> ("error out"=w440:errorcluster)  [unwired: 15 in, 2 out]
          }
        }
        n183 = call "DAQ_channels.vi"("error in"=w400) -> ("error out"=w423:errorcluster, "task out"=w424:refnum<k21>)  [unwired: 9 in]
        n184 = call <vilib>:"DAQmx Start Task.vi"("task/channels in"=w424, "error in"=w423) -> ("task out"=w422:refnum<k21>, "error out"=w421:errorcluster)  [unwired: 12 in]
      }
      frame False {
        n185 = call-poly <vilib>:"DAQmx Read.vi"("task/channels in"=w496, "number of samples per channel"=1000, "error in"=w498) -> ("task out"=w493:refnum<k21>, "data"=w484:waveform(dbl)[], "error out"=w497:errorcluster)  [unwired: 10 in]
        n186 = Enqueue Element(queue=w495, element=w484, error in (no error)=w497) -> (queue out=w494:refnum<queue>, error out=w490:errorcluster)  [unwired: 2 out]
        n187 = Enqueue Element(queue=w491, element=w484, error in (no error)=w490) -> (queue out=w489:refnum<queue>, error out=w488:errorcluster)  [unwired: 2 out]
        n188 = Enqueue Element(queue=w486, element=w484, error in (no error)=w488) -> (queue out=w485:refnum<queue>, error out=w487:errorcluster)  [unwired: 2 out]
      }
    }
    n189 = Unbundle By Name(w384) -> ("code"=w386:i32, "source"=w385:string)
    n190 = call <vilib>:"Simple Error Handler.vi"("error code (no error:0)"=w386, "error source (\" \")"=w385, "type of dialog (OK msg:1)"=w378, "error in (no error)"=w384) -> ("error out"=w379:errorcluster)  [unwired: 1 in, 4 out]
    "Numeric 2" <- w389
    "stop Ind" <- "stop"
  }
  n191 = call <vilib>:"DAQmx Stop Task.vi"("task/channels in"=w27, "error in"=w39) -> ("task out"=w37:refnum<k21>, "error out"=w38:errorcluster)  [unwired: 12 in]
  n192 = call <vilib>:"DAQmx Clear Task.vi"("task in"=w37, "error in"=w38) -> ("error out"=w33:errorcluster)  [unwired: 13 in]
  n193 = Merge Errors(w23, w28, w32, w33, w12) -> (w29:errorcluster)
  n194 = flat-sequence {
    tunnel: w31 -> [w503]
    tunnel: [w503] -> w30
    tunnel: w29 -> [w502]
    tunnel: [w502] -> w17
    tunnel: w19 -> [w500]
    tunnel: [w500] -> w18
    tunnel: [w499] -> w6
    tunnel: w5 -> [w499]
    frame #0 {
      n195 = local write "stop"(FALSE ("create if not found? (T)")) -> ()
    }
  }
  n196 = Release Queue(queue=w18, error in (no error)=w17) -> (error out=w16:errorcluster)  [unwired: 1 in, 2 out]
  n197 = Release Queue(queue=w30, error in (no error)=w16) -> (error out=w8:errorcluster)  [unwired: 1 in, 2 out]
  n198 = Release Queue(queue=w6, error in (no error)=w8) -> (error out=w7:errorcluster)  [unwired: 1 in, 2 out]
  n199 = Unbundle By Name(w7) -> ("code"=w43:i32, "source"=w42:string)
  n200 = call <vilib>:"Simple Error Handler.vi"("error code (no error:0)"=w43, "error source (\" \")"=w42, "error in (no error)"=w7) -> ("error?"=w34:bool, "error out"=w35:errorcluster, "message"=w36:string)  [unwired: 2 in, 2 out]
  n201 = call "Display Message to User"("error in (no error)"=w35, "Enable"=w34, "Message"=w36) -> ()  [unwired: 7 in, 2 out]
